vi "Pressure_Multiplexer_Server.vi"(5 "DAQ Trigger Port":refnum<visa-resource-name>="COM100", 6 "Current Block No":i32, 7 "DAQ Tigger Control?":bool, 8 "Time per Block (s)":dbl=100.0 format="%_4f", 9 "Trigger mode":T3, 10 "setup":T2=enum."Show Setup", 11 "Device port info":T1[](array[typedef])) -> (0 "DAQ Error":errorcluster, 3 "Array of Data Clusters":T4[](array[typedef]))   [LabVIEW 2020]
uses:
  Controls/Fixed sampling rate Data Cluster.ctl
  Controls/Trigger_Mode.ctl
  Controls/Setup.ctl
  Device ID port info.ctl
  <vilib>/Instr/_visa.llb/VISA Find Search Mode.ctl
  Globals/Meas_global.vi
  Pressure_Multiplexer_Server_Global.vi
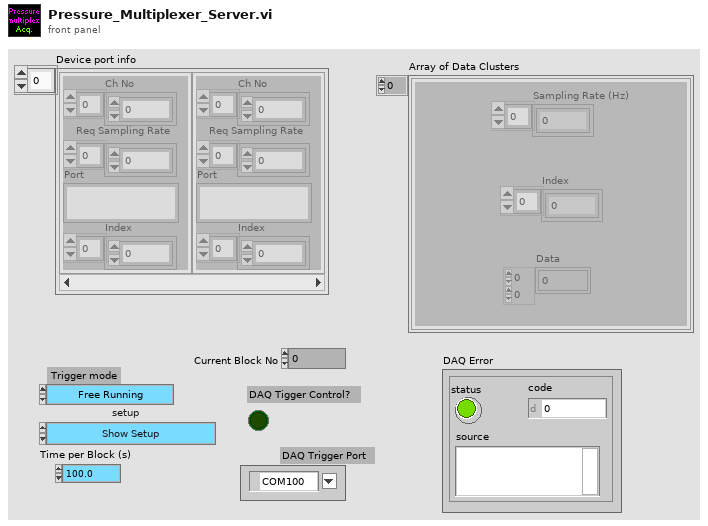
[diagram p1: front panel]
types:
  T1 = typedef "Device ID port info.ctl" = cluster{"Ch No":i16[], "Req Sampling Rate":dbl[], "Port":string, "Index":i32[]}
  T2 = typedef "Setup.ctl" = enum16{"Run Program", "Show Setup", "Save Current Setup", "Setup Front Panel"}
  T3 = typedef "Trigger_Mode.ctl" = enum16{"Free Running", "Start on Trigger", "Trigger Every Block", "Trigger Every Sample"}
  T4 = typedef "Fixed sampling rate Data Cluster.ctl" = cluster{"Sampling Rate (Hz)":dbl[], "Data":dbl[][], "Index":i32[]}
  T5 = typedef "Rendezvous RefNum" = refnum<k1>
  T6 = typedef "VISA Find Search Mode.ctl" = u32
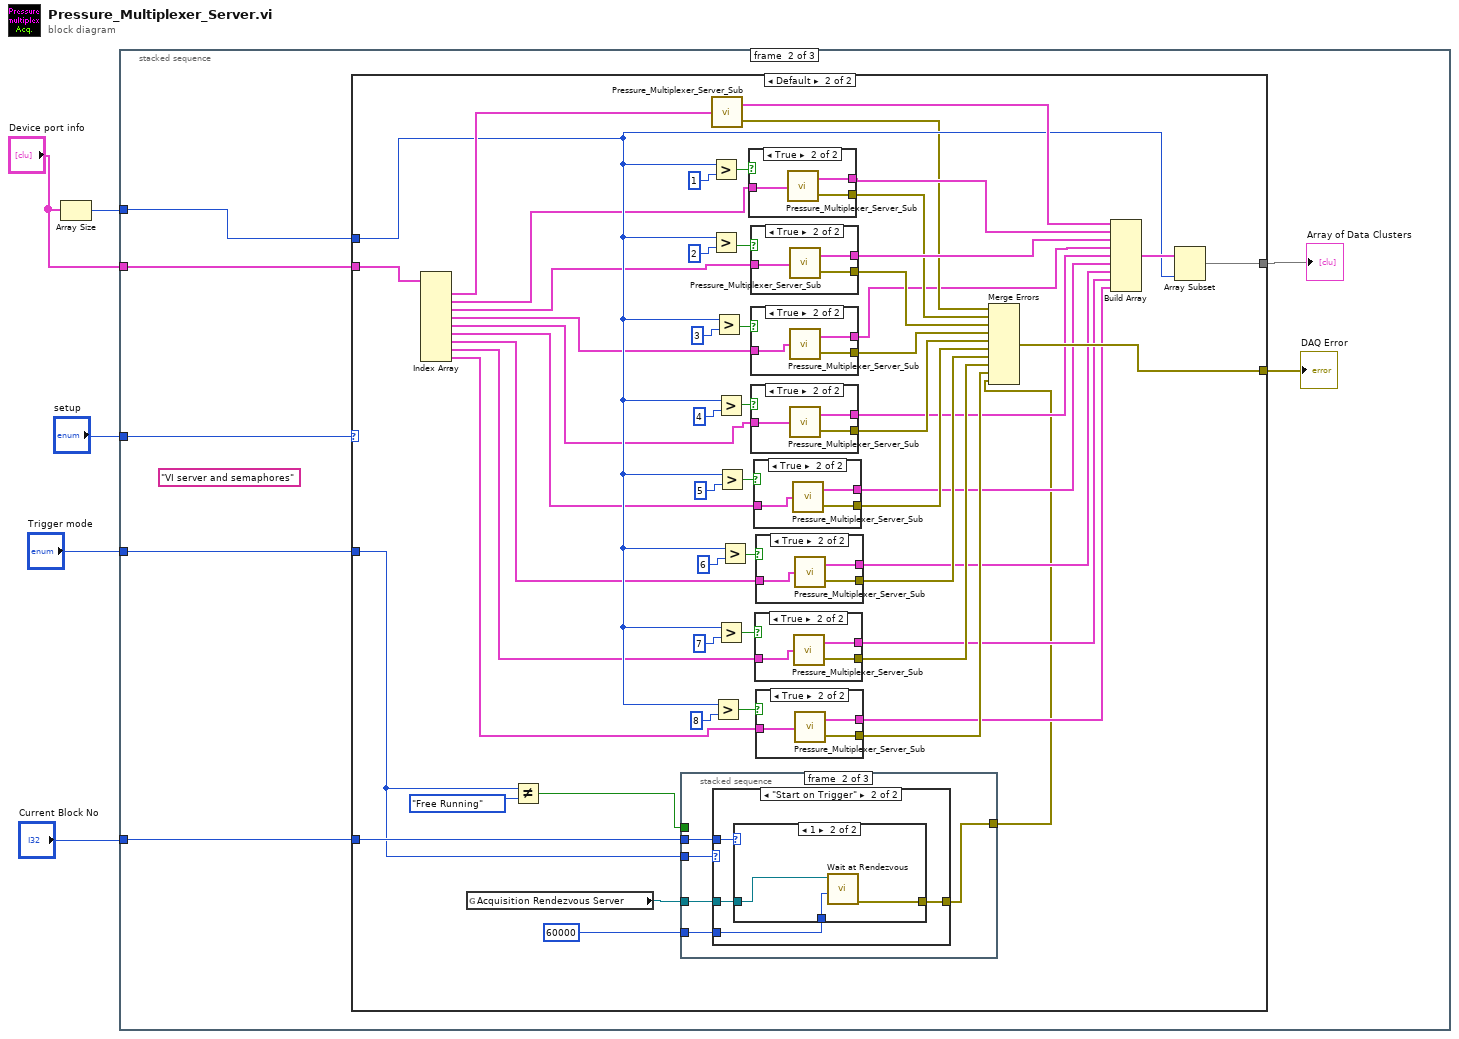
[diagram p0: block diagram]
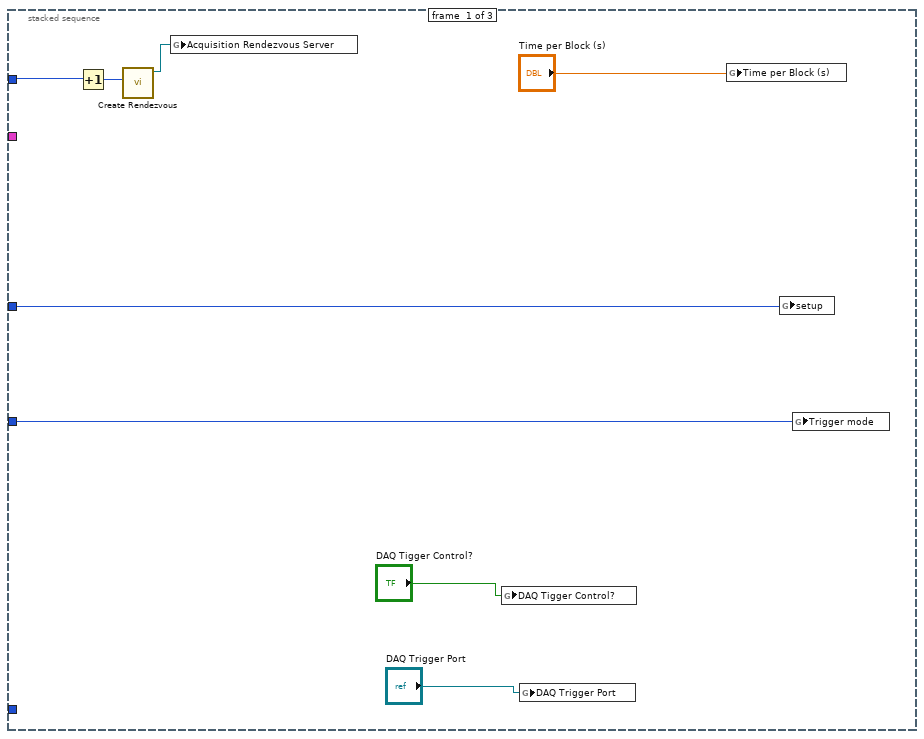
[diagram p2: hidden frame]
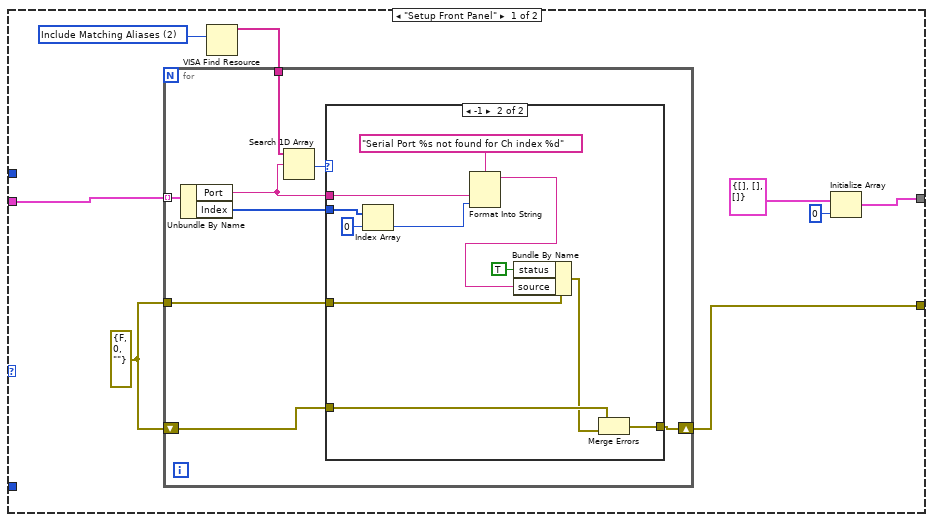
[diagram p3: hidden frame]
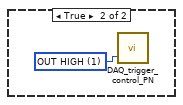
[diagram p6: hidden frame]
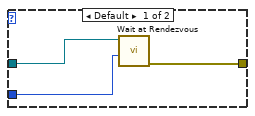
[diagram p7: hidden frame]
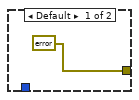
[diagram p8: hidden frame]
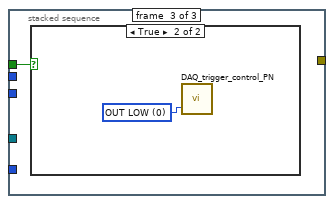
[diagram p9: hidden frame]
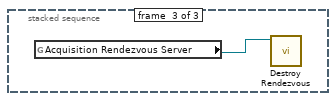
[diagram p19: hidden frame]
diagram:
  n1 = Array Size(array="Device port info") -> (size(s)=w3:i32)
  n2 = stacked-sequence {
    tunnel: "setup" -> [w12 w18 _]
    tunnel: "Device port info" -> [_ w17 _]
    tunnel: w3 -> [w10 w16 _]
    tunnel: "Trigger mode" -> [w8 w15 _]
    tunnel: "Current Block No" -> [_ w14 _]
    frame #0 {
      n3 = Increment(x=w10) -> (x+1=w11:i32)
      n4 = call <vilib>:"Create Rendezvous.vi"("size (2)"=w11) -> ("rendezvous"=w9:T5)  [unwired: 4 in, 2 out]
      n5 = global write "Pressure_Multiplexer_Server_Global.vi" "Acquisition Rendezvous Server"(w9) -> ()
      n6 = global write "Meas_global.vi" "DAQ Tigger Control?"("DAQ Tigger Control?") -> ()
      n7 = global write "Meas_global.vi" "DAQ Trigger Port"("DAQ Trigger Port") -> ()
      n8 = global write "Pressure_Multiplexer_Server_Global.vi" "Time per Block (s)"("Time per Block (s)") -> ()
      n9 = global write "Pressure_Multiplexer_Server_Global.vi" "setup"(w12) -> ()
      n10 = global write "Pressure_Multiplexer_Server_Global.vi" "Trigger mode"(w8) -> ()
    }
    frame #1 {
      (unwired) "VI server and semaphores"
      n11 = case shown="Default" w18 {
        tunnel: w17 -> [w28 w103]
        tunnel: w16 -> [_ w90]
        tunnel: [w27 w96] -> w20
        tunnel: [w22 w89] -> w19
        tunnel: w15 -> [_ w62]
        tunnel: w14 -> [_ w63]
        frame "Setup Front Panel" {
          w26 = T6 2 items=["Canonical Names Only"=0, "Aliases Only"=1, "Include Matching Aliases"=2, "Include All Aliases"=4] ("Search Mode")
          w24 = errorcluster {"status"=FALSE, "code"=0, "source"=""} ("error IO")
          n12 = VISA Find Resource(10:w26) -> (3:w25:string[])  [unwired: 1 in, 3 out]
          n13 = for {
            tunnel: w28 -> [w36] mode=indexing
            shift-right: [w34] -> w27
            shift-left: w24 -> [w35]
            tunnel: w25 -> [w33]
            tunnel: w24 -> [w31]
            n14 = Unbundle By Name(w36) -> ("Port"=w30:string, "Index"=w29:i32[])
            n15 = Search 1D Array(1D array=w33, element=w30) -> (index of element=w32:i32)  [unwired: 1 in]
            n16 = case shown="-1" w32 {
              tunnel: w35 -> [w37 w47]
              tunnel: [w37 w48] -> w34
              tunnel: w31 -> [_ w44]
              tunnel: w30 -> [_ w43]
              tunnel: w29 -> [_ w41]
              frame 0, Default {
              }
              frame -1 {
                n17 = Index Array(array=w41, index=0) -> (element=w38:i32)
                n18 = Format Into String(format string="Serial Port %s not found for Ch index %d", w43, w38) -> (resulting string=w39:string)  [unwired: 2 in, 1 out]
                n19 = Bundle By Name(cluster=w44, "status"=TRUE, "source"=w39) -> (w45:errorcluster)
                n20 = Merge Errors(w47, w45) -> (w48:errorcluster)
              }
            }
          }
          n21 = Initialize Array(T4 {"Sampling Rate (Hz)"=[], "Data"=[], "Index"=[]} ("Data Cluster"), 0 ("dimension size")) -> (w22:T4[])
        }
        frame Default {
          n22 = Index Array(array=w103) -> (element #1=w95:T1, element #2=w87:T1, element #3=w83:T1, element #4=w52:T1, element #5=w51:T1, element #6=w50:T1, element #7=w53:T1, element #8=w54:T1, element #9=w81:T1)  [unwired: 9 in]
          n23 = global read "Pressure_Multiplexer_Server_Global.vi" "Acquisition Rendezvous Server"() -> (w60:T5)
          n24 = Not Equal?(x=w62, y=Trigger_Mode."Free Running" ("Trigger mode")) -> (x != y?=w64:bool)
          n25 = stacked-sequence {
            tunnel: [_ w109 _] -> w49
            tunnel: w64 -> [w104 _ w122]
            tunnel: w63 -> [_ w110 _]
            tunnel: w62 -> [_ w108 _]
            tunnel: 60000 ("ms timeout (-1)") -> [_ w107 _]
            tunnel: w60 -> [_ w106 _]
            frame #0 {
              n26 = case shown="False" w104 {
                frame False {
                }
                frame True {
                  w105 = u8 1 items=["OUT LOW", "OUT HIGH", "IN READ"] ("Action")
                  n27 = call "DAQ_trigger_control_PN.vi"("Action"=w105) -> ()  [unwired: 1 in, 3 out]
                }
              }
            }
            frame #1 {
              n28 = case shown="\"Start on Trigger\"" w108 {
                tunnel: w110 -> [_ w117]
                tunnel: [w113 w116] -> w109
                tunnel: w107 -> [w112 w115]
                tunnel: w106 -> [w111 w114]
                frame Default {
                  n29 = call <vilib>:"Wait at Rendezvous.vi"("ms timeout (-1)"=w112, "rendezvous"=w111) -> ("error out"=w113:errorcluster)  [unwired: 3 in, 2 out]
                }
                frame "Start on Trigger" {
                  n30 = case shown="1" w117 {
                    tunnel: [errorcluster {"status"=FALSE, "code"=0, "source"=""} ("error out") w121] -> w116
                    tunnel: w115 -> [_ w120]
                    tunnel: w114 -> [_ w119]
                    frame Default {
                    }
                    frame 1 {
                      n31 = call <vilib>:"Wait at Rendezvous.vi"("ms timeout (-1)"=w120, "rendezvous"=w119) -> ("error out"=w121:errorcluster)  [unwired: 3 in, 2 out]
                    }
                  }
                }
              }
            }
            frame #2 {
              n32 = case shown="True" w122 {
                frame False {
                }
                frame True {
                  w123 = u8 0 items=["OUT LOW", "OUT HIGH", "IN READ"] ("Action")
                  n33 = call "DAQ_trigger_control_PN.vi"("Action"=w123) -> ()  [unwired: 1 in, 3 out]
                }
              }
            }
          }
          n34 = Greater?(x=w90, y=1) -> (0:w88:bool)
          n35 = Greater?(x=w90, y=2) -> (0:w84:bool)
          n36 = call "Pressure_Multiplexer_Server_Sub.vi"("Single Pres Multiplexer"=w95) -> ("Data Cluster"=w92:T4, "DAQ Error"=w72:errorcluster)
          n37 = Greater?(x=w90, y=8) -> (0:w82:bool)
          n38 = Greater?(x=w90, y=3) -> (0:w59:bool)
          n39 = Greater?(x=w90, y=4) -> (0:w58:bool)
          n40 = Greater?(x=w90, y=7) -> (0:w55:bool)
          n41 = Greater?(x=w90, y=5) -> (0:w57:bool)
          n42 = Greater?(x=w90, y=6) -> (0:w56:bool)
          n43 = case shown="True" w88 {
            tunnel: w87 -> [_ w144]
            tunnel: [_ w143] -> w73
            tunnel: [_ w142] -> w86
            frame False {
            }
            frame True {
              n44 = call "Pressure_Multiplexer_Server_Sub.vi"("Single Pres Multiplexer"=w144) -> ("Data Cluster"=w142:T4, "DAQ Error"=w143:errorcluster)
            }
          }
          n45 = case shown="True" w84 {
            tunnel: w83 -> [_ w141]
            tunnel: [_ w140] -> w74
            tunnel: [_ w139] -> w85
            frame False {
            }
            frame True {
              n46 = call "Pressure_Multiplexer_Server_Sub.vi"("Single Pres Multiplexer"=w141) -> ("Data Cluster"=w139:T4, "DAQ Error"=w140:errorcluster)
            }
          }
          n47 = case shown="True" w59 {
            tunnel: [_ w138] -> w80
            tunnel: [_ w137] -> w71
            tunnel: w52 -> [_ w136]
            frame False {
            }
            frame True {
              n48 = call "Pressure_Multiplexer_Server_Sub.vi"("Single Pres Multiplexer"=w136) -> ("Data Cluster"=w137:T4, "DAQ Error"=w138:errorcluster)
            }
          }
          n49 = case shown="True" w58 {
            tunnel: [_ w135] -> w79
            tunnel: [_ w134] -> w70
            tunnel: w51 -> [_ w133]
            frame False {
            }
            frame True {
              n50 = call "Pressure_Multiplexer_Server_Sub.vi"("Single Pres Multiplexer"=w133) -> ("Data Cluster"=w134:T4, "DAQ Error"=w135:errorcluster)
            }
          }
          n51 = case shown="True" w57 {
            tunnel: [_ w132] -> w78
            tunnel: [_ w131] -> w69
            tunnel: w50 -> [_ w130]
            frame False {
            }
            frame True {
              n52 = call "Pressure_Multiplexer_Server_Sub.vi"("Single Pres Multiplexer"=w130) -> ("Data Cluster"=w131:T4, "DAQ Error"=w132:errorcluster)
            }
          }
          n53 = case shown="True" w55 {
            tunnel: [_ w126] -> w76
            tunnel: [_ w125] -> w67
            tunnel: w54 -> [_ w124]
            frame False {
            }
            frame True {
              n54 = call "Pressure_Multiplexer_Server_Sub.vi"("Single Pres Multiplexer"=w124) -> ("Data Cluster"=w125:T4, "DAQ Error"=w126:errorcluster)
            }
          }
          n55 = case shown="True" w56 {
            tunnel: [_ w129] -> w77
            tunnel: [_ w128] -> w68
            tunnel: w53 -> [_ w127]
            frame False {
            }
            frame True {
              n56 = call "Pressure_Multiplexer_Server_Sub.vi"("Single Pres Multiplexer"=w127) -> ("Data Cluster"=w128:T4, "DAQ Error"=w129:errorcluster)
            }
          }
          n57 = case shown="True" w82 {
            tunnel: w81 -> [_ w147]
            tunnel: [_ w146] -> w75
            tunnel: [_ w145] -> w66
            frame False {
            }
            frame True {
              n58 = call "Pressure_Multiplexer_Server_Sub.vi"("Single Pres Multiplexer"=w147) -> ("Data Cluster"=w145:T4, "DAQ Error"=w146:errorcluster)
            }
          }
          n59 = Merge Errors(w72, w73, w74, w80, w79, w78, w77, w76, w75, w49) -> (w96:errorcluster)
          n60 = Build Array(w92, w86, w85, w71, w70, w69, w68, w67, w66) -> (w91:T4[])
          n61 = Array Subset(array=w91, length=w90) -> (w89:T4[])  [unwired: 1 in]
        }
      }
      "DAQ Error" <- w20
      "Array of Data Clusters" <- w19
    }
    frame #2 {
      n62 = global read "Pressure_Multiplexer_Server_Global.vi" "Acquisition Rendezvous Server"() -> (w148:T5)
      n63 = call <vilib>:"Destroy Rendezvous.vi"("rendezvous"=w148) -> ()  [unwired: 5 in, 2 out]
    }
  }
